vi "Set Protection Signal Incoming.vi"(6 "Protections":T1, 8 "error in (no error)":errorcluster, 9 "Protection Value":dbl, 10 "Frame.Data in":dbl[](array[numeric]), 11 "Protection Configuration in":T2 {"CRC Channels"."Data Type" items=["Signed", "Unsigned", "IEEE Float"]}) -> (0 "error out":errorcluster, 2 "Frame.Data out":dbl[](array[numeric]), 3 "Protection Configuration out":T2 {"CRC Channels"."Data Type" items=["Signed", "Unsigned", "IEEE Float"]})   [LabVIEW 2019, in "Protection and Counter Support Engine.lvlib"]
uses:
  Types/RT Protection Configuration.ctl
  Shared/Types/Protection Type.ctl
  Shared/Types/XNET Signal Configuration.ctl
  <vilib>/NI/NIVS Inline Async API/_Data Access Engine/Data Access Engine/Types/Write.DVR.ctl
  <vilib>/NI/NIVS Inline Async API/_Data Access Engine/Access Type Classes/Write/Write.lvclass
  <vilib>/NI/NIVS Inline Async API/_Data Access Engine/Access Type Classes/Write/Write.lvclass/Write.ctl
  <vilib>/NI/NIVS Inline Async API/_Data Access Engine/Data Access Engine/Methods/Write.Data.Buffer.vi
  <vilib>/NI/NIVS Inline Async API/_Data Access Engine/Access Type Classes/Write/Write.Buffer.vi
  Protection and Counter Support Engine.lvlib
  <vilib>/NI/NIVS Inline Async API/_Data Access Engine/Data Access Engine/Data Access Engine.lvclass
  Shared/Protection and Counter Support Shared.lvlib
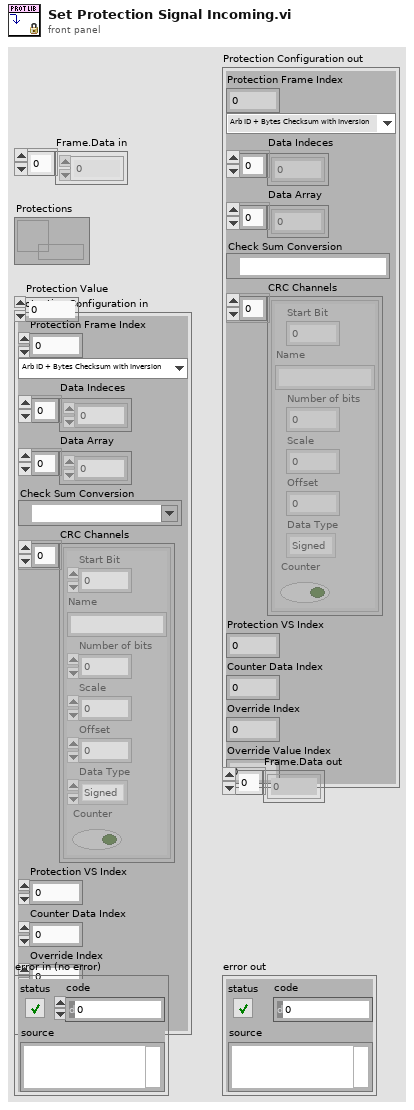
[diagram p1: front panel]
types:
  T1 = typedef "Data Access Engine.lvlib/Data Access Engine.lvclass/Write.DVR.ctl" = refnum<data-value>
  T2 = typedef "Protection and Counter Support Engine.lvlib/RT Protection Configuration.ctl" = cluster{"Protection Frame Index":i32, "Protection Type":T3, "Data Indeces":i32[], "Data Array":dbl[], "Check Sum Conversion":refnum<k21>, "CRC Channels":T4[], "Protection VS Index":i32, "Counter Data Index":i32, "Override Index":i32, "Override Value Index":i32}
  T3 = typedef "Protection and Counter Support Shared.lvlib/Protection Type.ctl" = enum16{"Arb ID + Bytes Checksum with Inversion", "Arb ID + Bytes CRC with Inversion", "Reversed Raw Signal Checksum with Inversion", "Concatenated Two's Compliment"}
  T4 = typedef "Protection and Counter Support Shared.lvlib/XNET Signal Configuration.ctl" = cluster{"Start Bit":i32, "Name":string, "Number of bits":i32, "Scale":dbl, "Offset":dbl, "Data Type":u32, "Counter":bool}
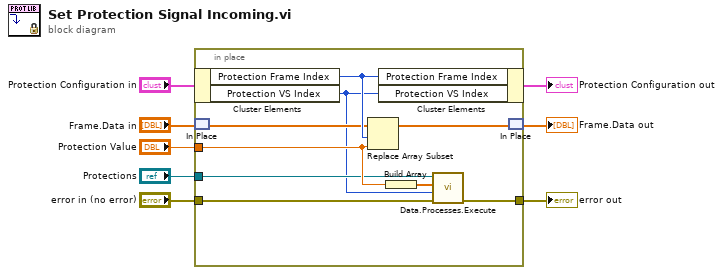
[diagram p0: block diagram]
diagram:
  n1 = in-place {
    in-place-border: "error in (no error)" -> [w17]
    in-place-border: [w16] -> w2
    in-place-border: "Protection Value" -> [w15]
    in-place-border: "Protections" -> [w14]
    n2 = in-place-cluster #1("Protection Configuration in") -> ("Protection Frame Index"=w13:i32, "Protection VS Index"=w10:i32)
    n3 = in-place-match #2("Frame.Data in") -> (w12:dbl[])
    n4 = Replace Array Subset(array=w12, new element=w15, index=w13) -> (w11:dbl[])
    n5 = in-place-cluster #1("Protection Frame Index"=w13, "Protection VS Index"=w10) -> (→"Protection Configuration out":T2)
    n6 = Build Array(w15) -> (w9:dbl[])
    n7 = call-poly <vilib>:"Data.Processes.Execute.vi"("error in (no error)"=w17, "Offset"=w10, "Values"=w9, "Ref"=w14) -> ("error out"=w16:errorcluster)  [unwired: 7 in]
    n8 = in-place-match #2(w11) -> (→"Frame.Data out":dbl[])
  }
  "error out" <- w2
